vi "FdxCmdTxUDPCreatePortCvi.vi"(8 "error in":errorcluster, 9 "UdpDescription":T1, 11 "InstrumentHandle":u32) -> (0 "error out":errorcluster, 2 "UdpHandle":u32, 3 "InstrumentHandle":u32)   [LabVIEW 2020, in "AIM664LV.lvlib"]
doc: "This function is used to create a port to transmit data from a specified UDP connection oriented port. Default settings after creation of the UDP port are:\n- UDP port enabled\n- Error injection: OFF\n- Skew (redundand mode only): 0 usec.\nTo change the settings of the UDP port the function AiFdxCmdTxUDPControl can be used. This function can be used only if transmitter is not running."
uses:
  AIM664LV.lvlib
  AFDX_LibraryAdmin/FdxGlobalDllPath.vi
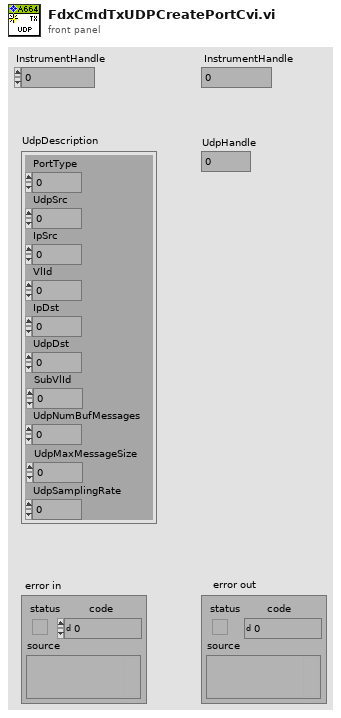
[diagram p1: front panel]
types:
  T1 = cluster{"PortType":u32, "UdpSrc":u32, "IpSrc":u32, "VlId":u32, "IpDst":u32, "UdpDst":u32, "SubVlId":u32, "UdpNumBufMessages":u32, "UdpMaxMessageSize":u32, "UdpSamplingRate":u32}
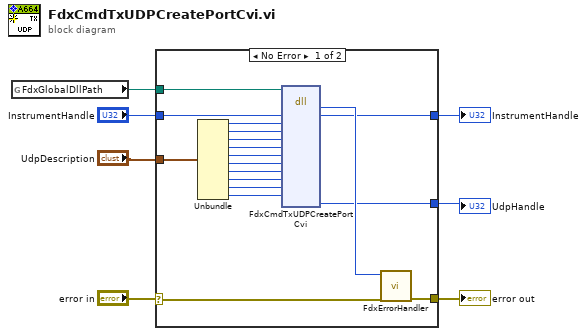
[diagram p0: block diagram]
diagram:
  n1 = global read "FdxGlobalDllPath.vi" "FdxGlobalDllPath"() -> (w5:path)
  n2 = case shown="No Error" "error in" {
    selector: "error in" -> [w24 w27]
    tunnel: [w25 w27] -> w7
    tunnel: w5 -> [w12 _]
    tunnel: [w11 w26] -> w4
    tunnel: "InstrumentHandle" -> [w10 w26]
    tunnel: [w9 _] -> w2
    tunnel: "UdpDescription" -> [w8 _]
    frame No Error {
      n3 = Unbundle(w8) -> ("PortType"=w22:u32, "UdpSrc"=w21:u32, "IpSrc"=w20:u32, "VlId"=w19:u32, "IpDst"=w18:u32, "UdpDst"=w17:u32, "SubVlId"=w16:u32, "UdpNumBufMessages"=w15:u32, "UdpMaxMessageSize"=w14:u32, "UdpSamplingRate"=w13:u32)
      n4 = dll-call lib="aim_fdx.19.dll" fn="FdxCmdTxUDPCreatePortCvi"(path in=w12, "InstrumentHandle"=w10, "PortType"=w22, "UdpSrc"=w21, "IpSrc"=w20, "VlId"=w19, "IpDst"=w18, "UdpDst"=w17, "SubVlId"=w16, "UdpNumBufMessages"=w15, "UdpMaxMessageSize"=w14, "UdpSamplingRate"=w13) -> ("status"=w23:i32, "InstrumentHandle"=w11:u32, "UdpHandle"=w9:u32)  [unwired: 12 in, 3 out]
      n5 = call "FdxErrorHandler.vi"("error in"=w24, "AIM Error"=w23) -> ("error out"=w25:errorcluster)  [unwired: 9 in]
    }
    frame Error {
    }
  }
  "error out" <- w7
  "InstrumentHandle" <- w4
  "UdpHandle" <- w2
